vi "LabToXYZ.vi"(1 "XrYrZr":dbl[](array[numeric]), 2 "L*a*b":dbl[](array[numeric])) -> (0 "XYZ":dbl[](array[numeric]))   [LabVIEW 2013]
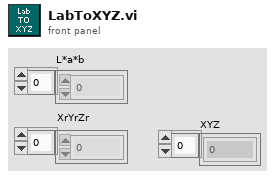
[diagram p1: front panel]
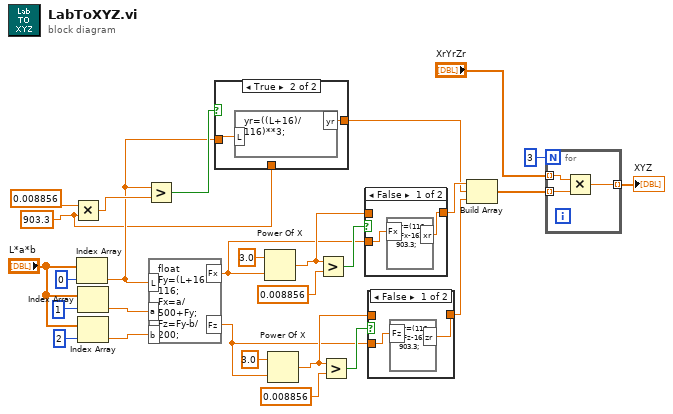
[diagram p0: block diagram]
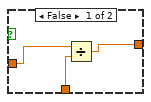
[diagram p2: hidden frame]
diagram:
  w8 = 903.3 ("y")
  n1 = Multiply(x=0.008856, y=w8) -> (x*y=w11:dbl)
  n2 = Index Array(array="L*a*b", index=0) -> (element=w9:dbl)
  n3 = Index Array(array="L*a*b", index=1) -> (element=w24:dbl)
  n4 = Index Array(array="L*a*b", index=2) -> (element=w23:dbl)
  n5 = Greater?(x=w9, y=w11) -> (0:w10:bool)
  n6 = formula code="float Fy=(L+16)/116;\nFx=a/500+Fy;\nFz=Fy-b/200;"("L"=w9, "a"=w24, "b"=w23) -> ("Fz"=w13:dbl, "Fx"=w18:dbl)
  n7 = case shown="True" w10 {
    tunnel: w9 -> [w31 w33]
    tunnel: [w29 w32] -> w6
    tunnel: w8 -> [w30 _]
    frame False {
      n8 = Divide(x=w31, y=w30) -> (x/y=w29:dbl)
    }
    frame True {
      n9 = formula code="yr=((L+16)/116)**3;"("L"=w33) -> ("yr"=w32:dbl)
    }
  }
  n10 = Power Of X(1:w18, 2:3.0 ("y")) -> (0:w19:dbl)
  n11 = Power Of X(1:w13, 2:3.0 ("y")) -> (0:w14:dbl)
  n12 = Greater?(x=w19, y=0.008856) -> (0:w20:bool)
  n13 = Greater?(x=w14, y=0.008856) -> (0:w15:bool)
  n14 = case shown="False" w20 {
    tunnel: w19 -> [_ w36]
    tunnel: [w34 w36] -> w7
    tunnel: w18 -> [w35 _]
    frame False {
      n15 = formula code="xr=(116*Fx-16)/903.3;"("Fx"=w35) -> ("xr"=w34:dbl)
    }
    frame True {
    }
  }
  n16 = case shown="False" w15 {
    tunnel: w14 -> [_ w39]
    tunnel: [w37 w39] -> w5
    tunnel: w13 -> [w38 _]
    frame False {
      n17 = formula code="zr=(116*Fz-16)/903.3;"("Fz"=w38) -> ("zr"=w37:dbl)
    }
    frame True {
    }
  }
  n18 = Build Array(w7, w6, w5) -> (w2:dbl[])
  n19 = for {
    N: 3 -> [_]
    tunnel: "XrYrZr" -> [w41] mode=indexing
    tunnel: w2 -> [w42] mode=indexing
    tunnel: [w40] -> w1 mode=indexing
    n20 = Multiply(x=w41, y=w42) -> (x*y=w40:dbl)
  }
  "XYZ" <- w1
